vi "Calculate Average.vi"(8 "error in":errorcluster, 10 "Function":string(combo), 11 "VISA resource name in":refnum<visa-resource-name>) -> (0 "error out":errorcluster, 2 "Value":dbl, 3 "VISA resource name out":refnum<visa-resource-name>)   [LabVIEW 2021, in "Keysight U1282A.lvlib"]
doc: "El comando de calculo promedio (CALC:AVER) regresa un registro din;amico de función en específico: Maximum - Máximo valor registrado\nMinimum - Mínimo valor registrado\nAverage - Valor promedio registrado\nPresent - Valor actual registrado\nCount - Valor del contador del modo promedio"
uses:
  Keysight U1282A.lvlib
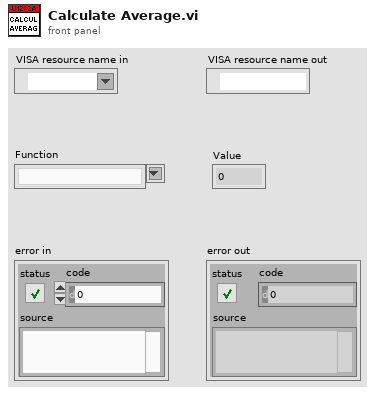
[diagram p1: front panel]
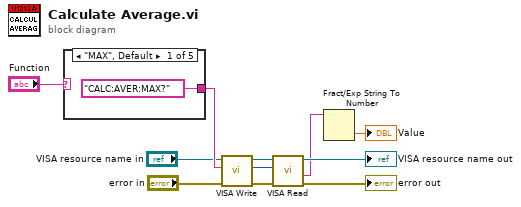
[diagram p0: block diagram]
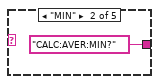
[diagram p2: hidden frame]
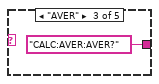
[diagram p3: hidden frame]
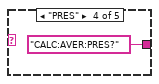
[diagram p4: hidden frame]
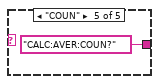
[diagram p5: hidden frame]
diagram:
  n1 = case shown="\"MAX\", Default" "Function" {
    tunnel: ["CALC:AVER:MAX?" "CALC:AVER:MIN?" "CALC:AVER:AVER?" "CALC:AVER:PRES?" "CALC:AVER:COUN?"] -> w10
    frame "MAX", Default {
    }
    frame "MIN" {
    }
    frame "AVER" {
    }
    frame "PRES" {
    }
    frame "COUN" {
    }
  }
  n2 = call "VISA Write.vi"("error in"="error in", "SCPI command"=w10, "VISA resource in"="VISA resource name in") -> ("error out"=w5:errorcluster, "Bytes at Port out"=w6:u32, "VISA resource out"=w7:refnum<visa-resource-name>)  [unwired: 6 in]
  n3 = call "VISA Read.vi"("error in"=w5, "Bytes at Port in"=w6, "VISA resource in"=w7) -> ("error out"=→"error out":errorcluster, "Reading"=w2:string, "VISA resource out"=→"VISA resource name out":refnum<visa-resource-name>)  [unwired: 5 in, 1 out]
  n4 = Fract/Exp String To Number(string=w2) -> (number=→"Value":dbl)  [unwired: 3 in, 1 out]
